vi "3-2，3-4整合.vi"() -> ()   [LabVIEW 2018]
uses:
  <vilib>/measure/NI_MABase.lvlib
panel:
  in  "选项卡控件":enum32{"宏观比较", "细节比较"}(tab)
  out "复原信号比较":waveform(dbl)[](graph)
  out "量化噪声比较":waveform(dbl)[](graph)
  out "0值附近比较":waveform(dbl)[](graph)
  out "峰值附近比较":waveform(dbl)[](graph)
  out "非均匀量化信噪比(dB)":dbl
  out "均匀量化信噪比(dB)":dbl
  in  "参考电压Vref（V）":dbl=2.56
  in  "模拟信号参数":cluster{"频率(Hz)":dbl, "幅值(V)":dbl}={"频率(Hz)"=100.0, "幅值(V)"=2.5}
  # "通过参考电压自动计算量化阶"
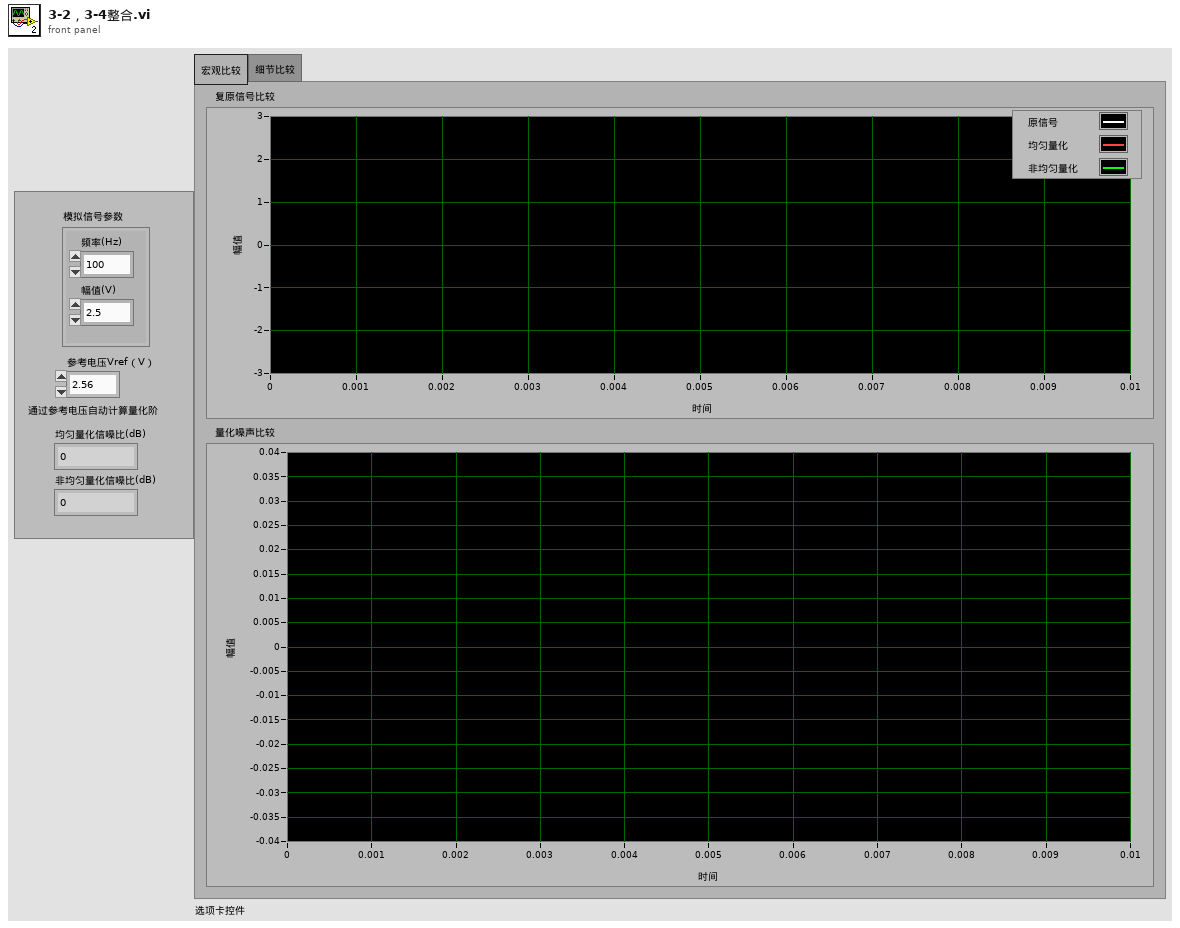
[diagram p1: front panel]
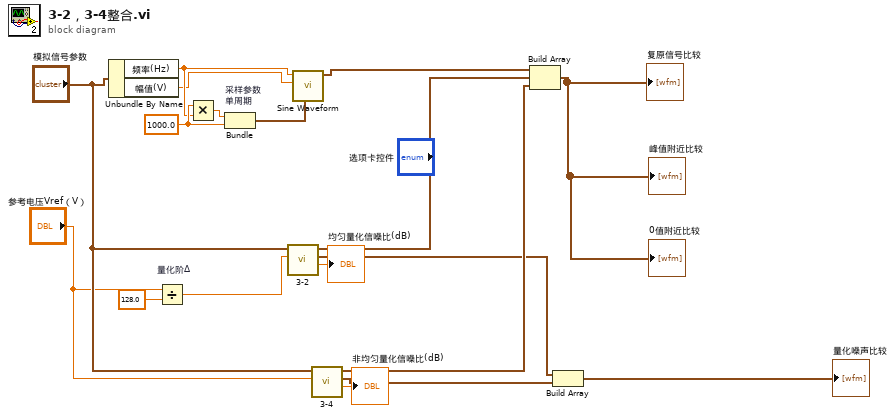
[diagram p0: block diagram]
diagram:
  w17 = 1000.0 ("x")
  n1 = Unbundle By Name("模拟信号参数") -> ("频率(Hz)"=w16:dbl, "幅值(V)"=w15:dbl)
  n2 = Divide "量化阶Δ"(x="参考电压Vref（V）", y=128.0) -> (x/y=w12:dbl)
  n3 = Multiply(x=w17, y=w16) -> (x*y=w18:dbl)
  n4 = Bundle "采样参数\n单周期"(w18, "x"=w17) -> (w14:cluster{dbl, "x":dbl})  [unwired: 1 in]
  n5 = call "3-2.vi"("量化阶Δ(V)"=w12, "模拟信号参数"="模拟信号参数") -> ("信噪比(dB)"=→"均匀量化信噪比(dB)":dbl, "量化噪声"=w5:waveform(dbl), "复原信号"=w8:waveform(dbl))  [unwired: 7 in]
  n6 = call <vilib>:"Sine Waveform.vi"("sampling info"=w14, "amplitude"=w15, "frequency"=w16) -> ("signal out"=w9:waveform(dbl))  [unwired: 7 in, 1 out]
  n7 = call "3-4.vi"("参考电压Vref（V）"="参考电压Vref（V）", "模拟信号参数"="模拟信号参数") -> ("信噪比(dB)"=→"非均匀量化信噪比(dB)":dbl, "量化噪声"=w4:waveform(dbl), "复原信号"=w7:waveform(dbl))  [unwired: 7 in]
  n8 = Build Array(w9, w8, w7) -> (→"复原信号比较" →"峰值附近比较" →"0值附近比较":waveform(dbl)[])
  n9 = Build Array(w5, w4) -> (→"量化噪声比较":waveform(dbl)[])
